vi "3.2.0 Kalman Control Cluster to Vector U.vi"(1 "Control Inputs U":T1) -> (0 "Real Matrix (Column Vector)":T2)   [LabVIEW 2010]
uses:
  <vilib>/Analysis/Matrix/Datatypes/RealMatrix.ctl
  <vilib>/Analysis/Matrix/Numeric/Conversions/Array To Matrix - RA.vi
  <vilib>/Analysis/Matrix/NI_Matrix.lvlib
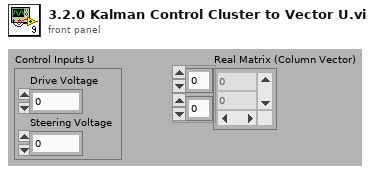
[diagram p1: front panel]
types:
  T1 = cluster{"Drive Voltage":dbl, "Steering Voltage":dbl}
  T2 = typedef "NI_Matrix.lvlib/RealMatrix.ctl" = dbl[][]
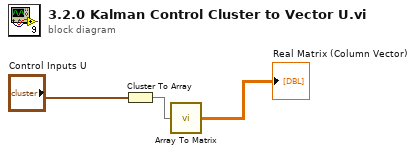
[diagram p0: block diagram]
diagram:
  n1 = Cluster To Array(cluster="Control Inputs U") -> (array=w2:dbl[])
  n2 = call-poly <vilib>:"Array To Matrix.vi"("Real 1D Array"=w2) -> ("Real Matrix (Column Vector)"=→"Real Matrix (Column Vector)":T2)
